vi "CFTS-Write state.vi"(8 "error in (no error)":errorcluster, 11 "Experiment info":T1) -> (0 "error out":errorcluster)   [LabVIEW 2020]
uses:
  CFTS-Experiment State.ctl
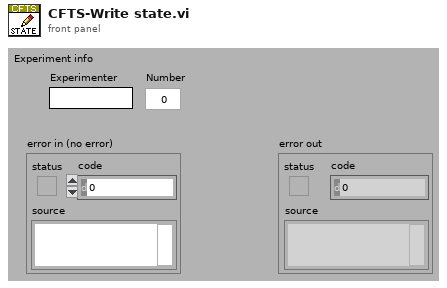
[diagram p1: front panel]
types:
  T1 = typedef "CFTS-Experiment State.ctl" = cluster{"Experimenter":string, "Number":u32, "Right":string, "Left":string, "Data Folder":path, "State File":path, "Version Info":string, "End Exposure Time":dbl, "Exposure Duration":string, "Run #":cluster{"CAP":i16, "ABR":i16, "DP":i16, "VsEP":i16, "MeasSeq":i16, "SubSeq":i16, "SFOAE":i16}}
  T2 = cluster{"CAP":i16, "ABR":i16, "DP":i16, "VsEP":i16, "MeasSeq":i16, "SubSeq":i16, "SFOAE":i16}
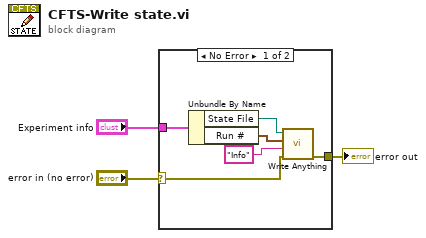
[diagram p0: block diagram]
diagram:
  n1 = case shown="No Error" "error in (no error)" {
    selector: "error in (no error)" -> [w5 w10]
    tunnel: "Experiment info" -> [w8 _]
    tunnel: [w6 w10] -> w2
    frame No Error {
      n2 = Unbundle By Name(w8) -> ("State File"=w9:path, "Run #"=w4:T2)
      n3 = call "Write Anything.vi"("Error In"=w5, "Section Name (Name of \"Anything\")"="Info" ("subkey"), "Anything"=w4, "Path (dialog)"=w9) -> ("Error Out"=w6:errorcluster)  [unwired: 6 in, 1 out]
    }
    frame Error {
    }
  }
  "error out" <- w2
